vi "Update Status.vi"(8 "error in":errorcluster, 9 "prettify json?":bool, 10 "Status":string) -> (0 "error out":errorcluster)   [LabVIEW 2024, in "GUI.lvlib"]
doc: "Report string to 'Status' string control\n_____\nCreated using DQMH Event Scripter 7.0.1.1316."
uses:
  GUI.lvlib
  Update Status Argument--cluster.ctl
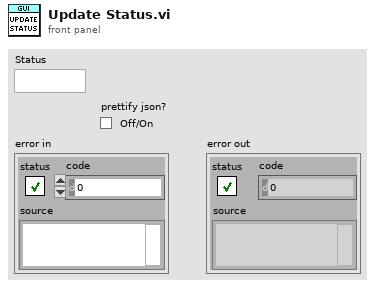
[diagram p1: front panel]
types:
  T1 = typedef "GUI.lvlib/Update Status Argument--cluster.ctl" = cluster{"Status":string, "Prettify JSON?":bool}
  T2 = typedef "GUI.lvlib/Request Events--cluster.ctl" = cluster{"Stop Module":refnum<user-event>, "Show Panel":refnum<user-event>, "Hide Panel":refnum<user-event>, "Get Module Execution Status":refnum<user-event>, "Show Diagram":refnum<user-event>, "Update Status":refnum<user-event>, "Private":cluster{"Get Waypoint":refnum<user-event>}}
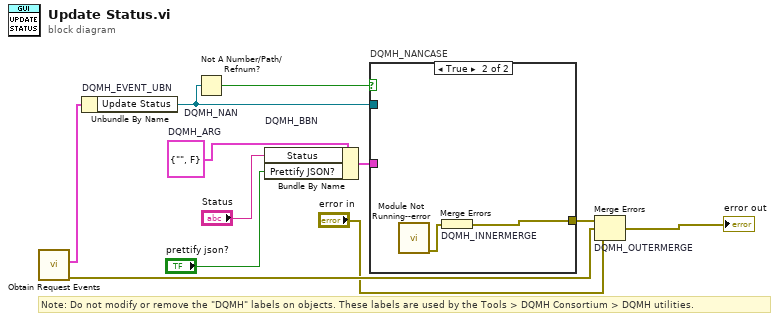
[diagram p0: block diagram]
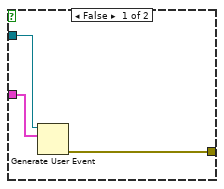
[diagram p2: hidden frame]
diagram:
  w6 = T1 {"Status"="", "Prettify JSON?"=FALSE}  # DQMH_ARG
  # "Note: Do not modify or remove the \"DQMH\" labels on objects. These labels are used by the Tools > DQMH Consortium > DQMH utilities."
  n1 = call "Obtain Request Events.vi"() -> ("error out"=w4:errorcluster, "GUI Request Events"=w3:T2)  [unwired: 10 in]
  n2 = Unbundle By Name "DQMH_EVENT_UBN"(w3) -> ("Update Status"=w8:refnum<user-event>)
  n3 = Not A Number/Path/Refnum? "DQMH_NAN"(number/path/refnum=w8) -> (NaN/Path/Refnum?=w9:bool)
  n4 = Bundle By Name "DQMH_BBN"(cluster=w6, "Status"="Status", "Prettify JSON?"="prettify json?") -> (w10:T1)
  n5 = case "DQMH_NANCASE" shown="True" w9 {
    tunnel: [w14 w16] -> w7
    tunnel: w8 -> [w13 _]
    tunnel: w10 -> [w12 _]
    frame False {
      n6 = Generate User Event(user event=w13, event data cluster=w12) -> (error out=w14:errorcluster)  [unwired: 2 in, 1 out]
    }
    frame True {
      n7 = call "Module Not Running--error.vi"() -> ("error out"=w15:errorcluster)  [unwired: 11 in]
      n8 = Merge Errors "DQMH_INNERMERGE"(w15) -> (w16:errorcluster)
    }
  }
  n9 = Merge Errors "DQMH_OUTERMERGE"(w7, w4, "error in") -> (→"error out":errorcluster)
